vi "Open Session - Options Set.vi"(8 "error in":errorcluster, 11 "Session in":refnum<class "Session.lvclass">) -> (0 "error out":errorcluster, 2 "Opened":bool, 3 "Session out":refnum<class "Session.lvclass">)   [LabVIEW 2015, in "Session.lvclass"]
uses:
  Session.lvclass
  C:/Program Files (x86)/WinSCP/WinSCPnet.dll
  Program Files (x86)/WinSCP/WinSCPnet.dll
  Session.lvclass/Session.ctl
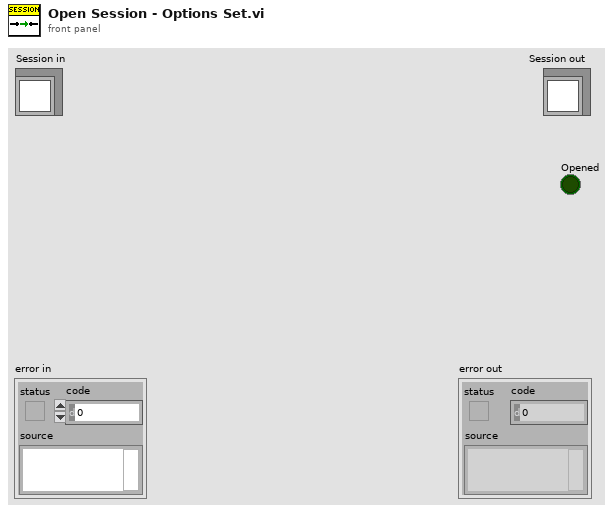
[diagram p1: front panel]
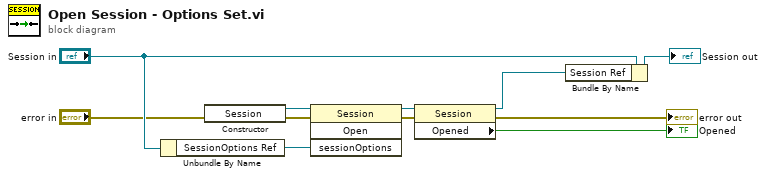
[diagram p0: block diagram]
diagram:
  n1 = Unbundle By Name("Session in") -> ("SessionOptions Ref"=w6:refnum<k24>)
  n2 = constructor class="Session"(error in="error in") -> (reference out=w11:refnum<k24>, error out=w10:errorcluster)  [unwired: 2 in, 1 out]
  n3 = invoke class="Session" method="Open"(reference=w11, error in=w10, "sessionOptions"=w6) -> (reference out=w9:refnum<k24>, error out=w8:errorcluster)  [unwired: 1 in, 2 out]
  n4 = property class="Session"(reference=w9, error in=w8) -> (reference out=w1:refnum<k24>, error out=→"error out":errorcluster, "Opened"=→"Opened":bool)
  n5 = Bundle By Name(cluster="Session in", "Session Ref"=w1) -> (→"Session out":refnum<class "Session.lvclass">)
